vi "Begin.vi"() -> (0 "error out":errorcluster)   [LabVIEW 2013]
doc: "Called before other user functions, this VI is expected to open initial I/O refnums, load in file data, and do all program initialization. Notice that the <B>error out</B> terminal is simply used for data flow. Wiring it to other structures or subVIs ensures that this VI runs first."
uses:
  <vilib>/Rock Robotics/WPI/SafetyOutput/WPI_SafetyOutputConfigMenu.ctl
  <vilib>/Rock Robotics/WPI/DriverStation/WPI_DriverStationRobotMode2.ctl
  <vilib>/Rock Robotics/WPI/Joystick/WPI_JoystickDeviceEnum.ctl
  <vilib>/Rock Robotics/SystemInterfaces/DIO/FPGA_DIOPWMChannel.ctl
  <vilib>/Rock Robotics/SystemInterfaces/Typedef/FPGA_TypedefAnalogModuleForGyro.ctl
  <vilib>/Rock Robotics/SystemInterfaces/AI/FPGA_AIGyroChannel.ctl
  <vilib>/Rock Robotics/SystemInterfaces/DIO/FPGA_DIOChannel.ctl
  <vilib>/Rock Robotics/SystemInterfaces/Typedef/FPGA_TypedefDigitalModule.ctl
  <vilib>/Rock Robotics/SystemInterfaces/DIO/FPGA_DIORelayChannel.ctl
  <vilib>/Rock Robotics/WPI/Solenoid/WPI_SolenoidChannel.ctl
  <vilib>/Rock Robotics/SystemInterfaces/AI/FPGA_AIChannel.ctl
  <vilib>/Rock Robotics/SystemInterfaces/Typedef/FPGA_TypedefAnalogModule.ctl
  <vilib>/Rock Robotics/SystemInterfaces/Typedef/FPGA_TypedefSolenoidModule.ctl
  <vilib>/Rock Robotics/WPI/Relay/WPI_RelayDirection.ctl
  <vilib>/Rock Robotics/WPI/Solenoid/WPI_SolenoidValue.ctl
  Robot Global Data.vi
  <vilib>/Rock Robotics/WPI/RobotDrive/WPI_RobotDriveOpen4MotorWithJaguar.vi
  <vilib>/Rock Robotics/WPI/Solenoid/WPI_SolenoidOpenDouble.vi
  <vilib>/Rock Robotics/WPI/Solenoid/WPI_SolenoidSetEnum.vi
  <vilib>/Rock Robotics/WPI/Compressor/WPI_CompressorGetSetRefNum.vi
  Custom VI's/Accelerometer/ADXL345 I2C Range.ctl
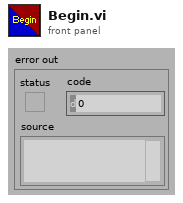
[diagram p1: front panel]
types:
  T1 = typedef "WPI_SolenoidValue.ctl" = enum16{"Off", "On", "Forward", "Reverse"}
  T2 = typedef "WPI_SolenoidChannel.ctl" = enum8{"Solenoid 1", "Solenoid 2", "Solenoid 3", "Solenoid 4", "Solenoid 5", "Solenoid 6", "Solenoid 7", "Solenoid 8", "Invalid"}
  T3 = typedef "FPGA_TypedefDigitalModule.ctl" = enum16{"Digital Module 1", "Digital Module 2"}
  T4 = typedef "WPI_RelayDirection.ctl" = enum16{"Both directions", "Forward only", "Reverse only"}
  T5 = typedef "FPGA_DIORelayChannel.ctl" = enum8{"Relay 1", "Relay 2", "Relay 3", "Relay 4", "Relay 5", "Relay 6", "Relay 7", "Relay 8", "Invalid"}
  T6 = typedef "FPGA_TypedefSolenoidModule.ctl" = enum16{"Solenoid Module 1", "Solenoid Module 2"}
  T7 = typedef "FPGA_AIChannel.ctl" = enum8{"AI 1", "AI 2", "AI 3", "AI 4", "AI 5", "AI 6", "AI 7", "AI 8", "Invalid"}
  T8 = typedef "FPGA_TypedefAnalogModule.ctl" = enum16{"Analog Module 1", "Analog Module 2"}
  T9 = typedef "FPGA_DIOChannel.ctl" = enum8{"DIO 1", "DIO 2", "DIO 3", "DIO 4", "DIO 5", "DIO 6", "DIO 7", "DIO 8", "DIO 9", "DIO 10", "DIO 11", "DIO 12", "DIO 13", "DIO 14", "Invalid"}
  T10 = typedef "WPI_JoystickDeviceEnum.ctl" = enum16{"USB 1", "USB 2", "USB 3", "USB 4", "Kinect 1", "Kinect 2"}
  T11 = typedef "FPGA_AIGyroChannel.ctl" = enum8{"AI 1", "AI 2", "Invalid"}
  T12 = typedef "FPGA_TypedefAnalogModuleForGyro.ctl" = enum16{"Analog Module 1"}
  T13 = typedef "FPGA_DIOPWMChannel.ctl" = enum8{"PWM 1", "PWM 2", "PWM 3", "PWM 4", "PWM 5", "PWM 6", "PWM 7", "PWM 8", "PWM 9", "PWM 10", "Invalid"}
  T14 = typedef "WPI_DriverStationRobotMode2.ctl" = enum16{"Autonomous Disabled", "Autonomous Enabled", "Teleop Disabled", "Teleop Enabled", "Timeout", "Finish", "Test Disabled", "Test Enabled"}
  T15 = typedef "WPI_SafetyOutputConfigMenu.ctl" = enum16{"Enable", "Disable"}
  T16 = typedef "WPI_GyroDevRef.ctl" = cluster{"DevStatus":errorcluster, "Analog Module":T8, "Analog Channel":T7, "Offset":dbl, "Gain (VoltsPerDegree/Second)":dbl}
  T17 = typedef "WPI_EncoderDevRef.ctl" = cluster{"DevStatus":errorcluster, "EncoderIndex":T18, "CounterIndex":T19, "DistancePerCount":dbl, "Decoding Type":T20}
  T18 = typedef "FPGA_EncoderIdx.ctl" = enum8{"Enc 0", "Enc 1", "Enc 2", "Enc 3", "Invalid"}
  T19 = typedef "FPGA_CounterCtrSystemIndex.ctl" = enum8{"Ctr 0", "Ctr 1", "Ctr 2", "Ctr 3", "Ctr 4", "Ctr 5", "Ctr 6", "Ctr 7", "Invalid"}
  T20 = typedef "WPI_EncoderType.ctl" = enum16{"1x", "2x", "4x"}
  T21 = cluster{"Motors[]":T17[], "DevStatus":errorcluster, "Max Speed[]":dbl[]}
  T22 = typedef "WPI_JoystickDevRef.ctl" = cluster{"Device":T10}
  T23 = typedef "WPI_RobotDriveDevRef.ctl" = cluster{"DevStatus":errorcluster, "Motors[]":T24[], "Square Inputs":bool, "Max Output":dbl, "Isochronous":bool}
  T24 = typedef "WPI_MotorControlDeviceRef.ctl" = cluster{"DeviceStatus":errorcluster, "Type":enum16{"PWM", "CAN"}, "PWM":cluster{"Digital Module":T3, "PWM Channel":T13, "DeadBand":T25}, "CAN":cluster{"Device Number":u8, "Control Mode":T26, "Semaphore":T27, "Max Vout":dbl}, "Invert":bool, "TransformRef":T28, "InvTransformRef":T28}
  T25 = typedef "WPI_PWMDeadband.ctl" = cluster{"Name":string, "maxPositivePwm":i32, "minPositivePwm":i32, "centerPwm":i32, "maxNegativePwm":i32, "minNegativePwm":i32, "angularRange":u16}
  T26 = typedef "WPI_CANJaguar_ControlMode.ctl" = enum8{"Percent VBus", "Current", "Speed", "Position", "Voltage"}
  T27 = typedef "Semaphore RefNum" = refnum<k1>
  T28 = typedef "WPI_PWMTransform_ConPane.ctl" = refnum<vi>
  T29 = typedef "ADXL345 I2C Range.ctl" = u8
  T30 = typedef "WPI_I2CDevRef.ctl" = cluster{"DevStatus":errorcluster, "Digital Module":T3, "Device Address":u8}
  T31 = typedef "WPI_SolenoidDevRef.ctl" = cluster{"DevStatus":errorcluster, "Solenoid Module":T6, "Forward Solenoid Channel":T2, "Reverse Solenoid Channel":T2}
  T32 = typedef "WPI_RelayDevRef.ctl" = cluster{"DevStatus":errorcluster, "Relay Channel":T5, "Digital Module":T3, "Relay Direction":T4}
  T33 = typedef "WPI_CompressorDevRef.ctl" = cluster{"DevStatus":errorcluster, "DigitalInputDevRef":T34, "RelayDevRef":T32}
  T34 = typedef "WPI_DigitalInputDevRef.ctl" = cluster{"DevStatus":errorcluster, "DIO Channel":T9, "Digital Module":T3}
  T35 = typedef "WPI_AnalogChannelDevRef.ctl" = cluster{"DevStatus":errorcluster, "Analog Module":T8, "Analog Channel":T7}
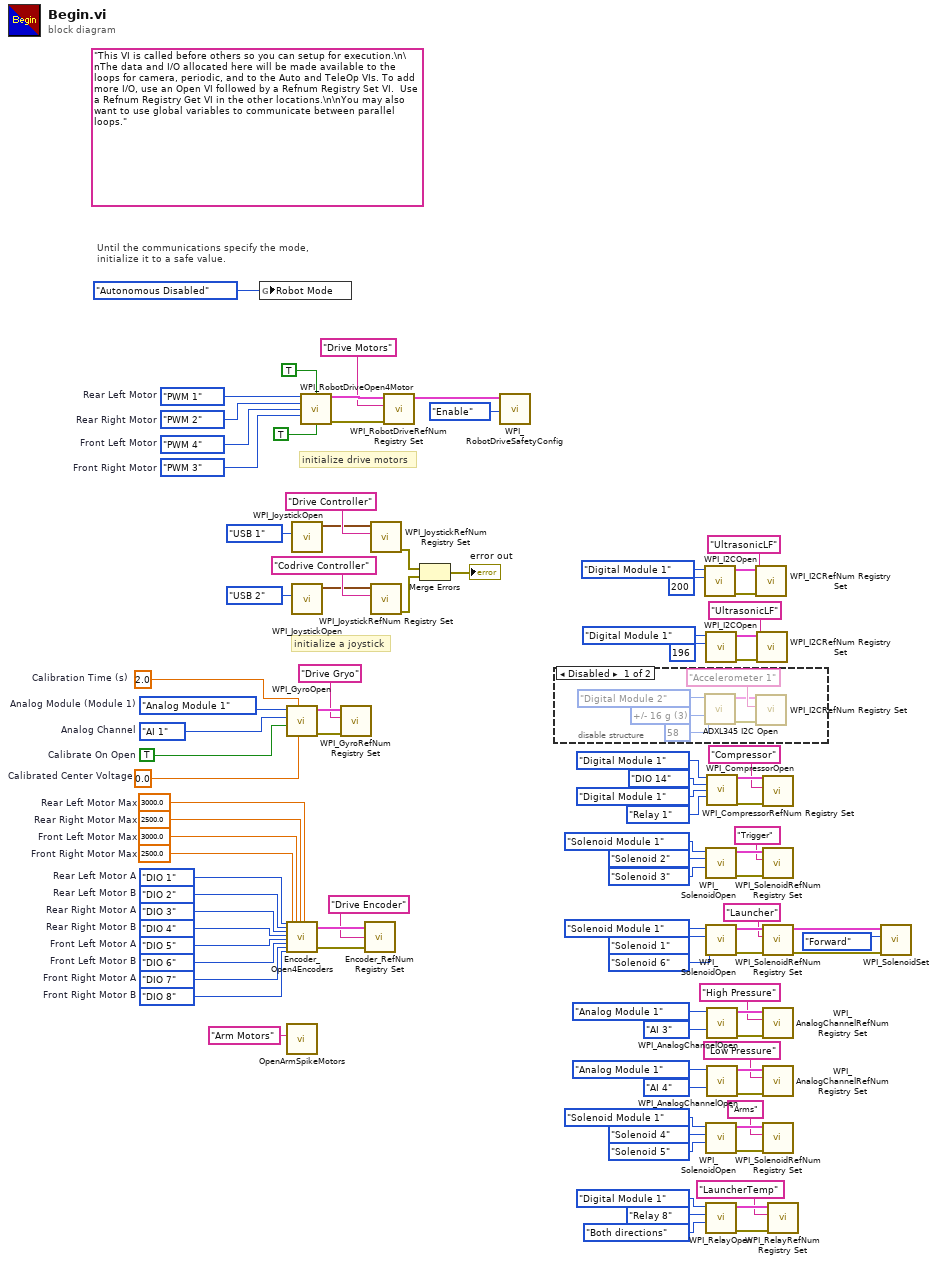
[diagram p0: block diagram]
diagram:
  w63 = 2500.0  # Front Right Motor Max
  w65 = 3000.0  # Front Left Motor Max
  w66 = 2500.0  # Rear Right Motor Max
  w67 = 3000.0  # Rear Left Motor Max
  w68 = FPGA_DIOChannel."DIO 8"  # Front Right Motor B
  w74 = FPGA_DIOChannel."DIO 7"  # Front Right Motor A
  w73 = FPGA_DIOChannel."DIO 6"  # Front Left Motor B
  w72 = FPGA_DIOChannel."DIO 5"  # Front Left Motor A
  w71 = FPGA_DIOChannel."DIO 4"  # Rear Right Motor B
  w70 = FPGA_DIOChannel."DIO 3"  # Rear Right Motor A
  w69 = FPGA_DIOChannel."DIO 2"  # Rear Left Motor B
  w64 = FPGA_DIOChannel."DIO 1"  # Rear Left Motor A
  w78 = 0.0  # Calibrated Center Voltage
  w79 = 2.0  # Calibration Time (s)
  w80 = TRUE  # Calibrate On Open
  w81 = FPGA_AIGyroChannel."AI 1"  # Analog Channel
  w82 = FPGA_TypedefAnalogModuleForGyro."Analog Module 1"  # Analog Module (Module 1)
  w86 = FPGA_DIOPWMChannel."PWM 3"  # Front Right Motor
  w87 = FPGA_DIOPWMChannel."PWM 4"  # Front Left Motor
  w88 = FPGA_DIOPWMChannel."PWM 2"  # Rear Right Motor
  w89 = FPGA_DIOPWMChannel."PWM 1"  # Rear Left Motor
  (unwired) "This VI is called before others so you can setup for execution.\n\nThe data and I/O allocated here will be made available to the loops for camera, periodic, and to the Auto and TeleOp VIs. To add more I/O, use an Open VI followed by a Refnum Registry Set VI.  Use a Refnum Registry Get VI in the other locations.\n\nYou may also want to use global variables to communicate between parallel loops."
  # "initialize a joystick"
  # "Until the communications specify the mode,\ninitialize it to a safe value."
  # "initialize drive motors"
  n1 = global write "Robot Global Data.vi" "Robot Mode"(WPI_DriverStationRobotMode2."Autonomous Disabled" ("Robot Mode")) -> ()
  n2 = call <vilib>:"WPI_GyroOpen.vi"("Calibrated Center Voltage"=w78, "Calibration Time (s)"=w79, "Calibrate On Open"=w80, "Analog Channel"=w81, "Analog Module (Module 1)"=w82) -> ("error out"=w84:errorcluster, "GyroDevRef"=w85:T16)  [unwired: 4 in, 1 out]
  n3 = call "Encoder_Open4Encoders.vi"("Rear Left Motor A"=w64, "Rear Left Motor B"=w69, "Rear Right Motor A"=w70, "Rear Right Motor B"=w71, "Front Left Motor A"=w72, "Front Left Motor B"=w73, "Front Right Motor A"=w74, "Front Right Motor B"=w68, "Front Right Motor Max"=w63, "Front Left Motor Max"=w65, "Rear Right Motor Max"=w66, "Rear Left Motor Max"=w67) -> ("RobotEncoderRef Out"=w76:T21, "error out"=w77:errorcluster)  [unwired: 14 in]
  n4 = call "OpenArmSpikeMotors.vi"("Name"="Arm Motors") -> ()  [unwired: 11 in]
  n5 = call <vilib>:"WPI_JoystickOpen.vi"("JoystickDevice"=WPI_JoystickDeviceEnum."USB 1") -> ("JoystickDevRef"=w91:T22)  [unwired: 10 in]
  n6 = call <vilib>:"WPI_JoystickOpen.vi"("JoystickDevice"=WPI_JoystickDeviceEnum."USB 2") -> ("JoystickDevRef"=w60:T22)  [unwired: 10 in]
  n7 = call-poly <vilib>:"WPI_RobotDriveOpen4Motor.vi"("Rear Left Motor"=w89, "Rear Right Motor Inverted"=TRUE, "Rear Right Motor"=w88, "Front Left Motor"=w87, "Front Right Motor"=w86, "Front Right Motor Inverted"=TRUE) -> ("RobotDriveDevRef"=w98:T23, "error out"=w96:errorcluster)  [unwired: 8 in]
  n8 = call <vilib>:"WPI_GyroRefNum Registry Set.vi"("error in (no error)"=w84, "refnum name"="Drive Gryo", "GyroDevRef"=w85) -> ()  [unwired: 7 in, 2 out]
  n9 = call "Encoder_RefNum Registry Set.vi"("error in (no error)"=w77, "refnum name"="Drive Encoder", "RobotEncoderRef"=w76) -> ()  [unwired: 2 out]
  n10 = call <vilib>:"WPI_JoystickRefNum Registry Set.vi"("refnum name"="Drive Controller", "JoystickDevRef"=w91) -> ("error out"=w57:errorcluster)  [unwired: 8 in, 1 out]
  n11 = call <vilib>:"WPI_JoystickRefNum Registry Set.vi"("refnum name"="Codrive Controller", "JoystickDevRef"=w60) -> ("error out"=w58:errorcluster)  [unwired: 8 in, 1 out]
  n12 = call <vilib>:"WPI_RobotDriveRefNum Registry Set.vi"("error in (no error)"=w96, "refnum name"="Drive Motors", "RobotDriveDevRef"=w98) -> ("RobotDriveDevRef"=w95:T23)  [unwired: 8 out]
  n13 = Merge Errors(w57, w58) -> (→"error out":errorcluster)
  n14 = call <vilib>:"WPI_RobotDriveSafetyConfig.vi"("mode"=WPI_SafetyOutputConfigMenu."Enable", "RobotDriveDevRef"=w95) -> ()  [unwired: 8 in, 2 out]
  n15 = disable-structure shown="Disabled" {
    frame Disabled {
      w101 = T29 3 items=["+/- 2 g", "+/- 4 g", "+/- 8 g", "+/- 16 g"] ("Range")
      n16 = call "ADXL345 I2C Open.vi"("Range"=w101, "Address"=u8 58, "DIO Module (Module 1)"=FPGA_TypedefDigitalModule."Digital Module 2") -> ("error out"=w104:errorcluster, "I2CDevRef"=w103:T30)  [unwired: 7 in]
      n17 = call <vilib>:"WPI_I2CRefNum Registry Set.vi"("error in (no error)"=w104, "refnum name"="Accelerometer 1", "I2CDevRef"=w103) -> ()  [unwired: 7 in, 2 out]
    }
    frame Enabled {
    }
  }
  n18 = call <vilib>:"WPI_I2COpen.vi"("Device Address"=u8 200, "Digital Module (Module 1)"=FPGA_TypedefDigitalModule."Digital Module 1") -> ("error out"=w47:errorcluster, "I2CDevRef"=w46:T30)  [unwired: 8 in]
  n19 = call <vilib>:"WPI_I2COpen.vi"("Device Address"=u8 196, "Digital Module (Module 1)"=FPGA_TypedefDigitalModule."Digital Module 1") -> ("error out"=w9:errorcluster, "I2CDevRef"=w8:T30)  [unwired: 8 in]
  n20 = call-poly <vilib>:"WPI_SolenoidOpen.vi"("Reverse Solenoid Channel"=WPI_SolenoidChannel."Solenoid 3", "Forward Solenoid Channel"=WPI_SolenoidChannel."Solenoid 2", "Solenoid Module (Module 1)"=FPGA_TypedefSolenoidModule."Solenoid Module 1") -> ("error out"=w38:errorcluster, "SolenoidDevRef"=w39:T31)  [unwired: 7 in]
  n21 = call-poly <vilib>:"WPI_SolenoidOpen.vi"("Reverse Solenoid Channel"=WPI_SolenoidChannel."Solenoid 6", "Forward Solenoid Channel"=WPI_SolenoidChannel."Solenoid 1", "Solenoid Module (Module 1)"=FPGA_TypedefSolenoidModule."Solenoid Module 1") -> ("error out"=w33:errorcluster, "SolenoidDevRef"=w34:T31)  [unwired: 7 in]
  n22 = call-poly <vilib>:"WPI_SolenoidOpen.vi"("Reverse Solenoid Channel"=WPI_SolenoidChannel."Solenoid 5", "Forward Solenoid Channel"=WPI_SolenoidChannel."Solenoid 4", "Solenoid Module (Module 1)"=FPGA_TypedefSolenoidModule."Solenoid Module 1") -> ("error out"=w21:errorcluster, "SolenoidDevRef"=w20:T31)  [unwired: 7 in]
  n23 = call <vilib>:"WPI_RelayOpen.vi"("Relay Direction"=WPI_RelayDirection."Both directions", "Relay Channel"=FPGA_DIORelayChannel."Relay 8", "Digital Module (Module 1)"=FPGA_TypedefDigitalModule."Digital Module 1") -> ("error out"=w14:errorcluster, "RelayDevRef"=w15:T32)  [unwired: 7 in]
  n24 = call <vilib>:"WPI_CompressorOpen.vi"("Pressure Switch Digital Module (Module 1)"=FPGA_TypedefDigitalModule."Digital Module 1", "Pressure Switch DIO Channel"=FPGA_DIOChannel."DIO 14", "Relay Digital Module (Module 1)"=FPGA_TypedefDigitalModule."Digital Module 1", "Relay Channel"=FPGA_DIORelayChannel."Relay 1") -> ("CompressorDevRef"=w54:T33, "error out"=w53:errorcluster)  [unwired: 10 in]
  n25 = call <vilib>:"WPI_AnalogChannelOpen.vi"("Analog Channel"=FPGA_AIChannel."AI 3", "Analog Module (Module 1)"=FPGA_TypedefAnalogModule."Analog Module 1") -> ("error out"=w30:errorcluster, "AIDeviceRef"=w31:T35)  [unwired: 8 in]
  n26 = call <vilib>:"WPI_AnalogChannelOpen.vi"("Analog Channel"=FPGA_AIChannel."AI 4", "Analog Module (Module 1)"=FPGA_TypedefAnalogModule."Analog Module 1") -> ("error out"=w25:errorcluster, "AIDeviceRef"=w26:T35)  [unwired: 8 in]
  n27 = call <vilib>:"WPI_I2CRefNum Registry Set.vi"("error in (no error)"=w47, "refnum name"="UltrasonicLF", "I2CDevRef"=w46) -> ()  [unwired: 7 in, 2 out]
  n28 = call <vilib>:"WPI_I2CRefNum Registry Set.vi"("error in (no error)"=w9, "refnum name"="UltrasonicLF", "I2CDevRef"=w8) -> ()  [unwired: 7 in, 2 out]
  n29 = call <vilib>:"WPI_CompressorRefNum Registry Set.vi"("error in (no error)"=w53, "refnum name"="Compressor", "CompressorDevRef"=w54) -> ()  [unwired: 7 in, 2 out]
  n30 = call <vilib>:"WPI_SolenoidRefNum Registry Set.vi"("error in (no error)"=w38, "refnum name"="Trigger", "SolenoidDevRef"=w39) -> ()  [unwired: 7 in, 2 out]
  n31 = call <vilib>:"WPI_SolenoidRefNum Registry Set.vi"("error in (no error)"=w33, "refnum name"="Launcher", "SolenoidDevRef"=w34) -> ("error out"=w1:errorcluster, "SolenoidDevRef"=w3:T31)  [unwired: 7 in]
  n32 = call <vilib>:"WPI_AnalogChannelRefNum Registry Set.vi"("error in (no error)"=w30, "refnum name"="High Pressure", "AIDeviceRef"=w31) -> ()  [unwired: 7 in, 2 out]
  n33 = call <vilib>:"WPI_AnalogChannelRefNum Registry Set.vi"("error in (no error)"=w25, "refnum name"="Low Pressure", "AIDeviceRef"=w26) -> ()  [unwired: 7 in, 2 out]
  n34 = call <vilib>:"WPI_SolenoidRefNum Registry Set.vi"("error in (no error)"=w21, "refnum name"="Arms", "SolenoidDevRef"=w20) -> ()  [unwired: 7 in, 2 out]
  n35 = call <vilib>:"WPI_RelayRefNum Registry Set.vi"("error in (no error)"=w14, "refnum name"="LauncherTemp", "RelayDevRef"=w15) -> ()  [unwired: 7 in, 2 out]
  n36 = call-poly <vilib>:"WPI_SolenoidSet.vi"("error in (no error)"=w1, "Value"=WPI_SolenoidValue."Forward", "SolenoidDevRef"=w3) -> ()  [unwired: 7 in, 2 out]
